vi "User Manage.vi"(11 "Name(\"\" to use uuid)":string="User Manage") -> ()   [LabVIEW 2020]
uses:
  <userlib>/_NEVSTOP/Communicable State Machine(CSM)/_Support/Priority Queue/Priority Queue.lvclass/Priority Queue.ctl
  <userlib>/_NEVSTOP/Communicable State Machine(CSM)/_Polymophic/Build Register Status Message.vi
  4963c333-465a-4436-b278-b1f160975599.vi
  7cf3f4c3-14bd-4f57-b2e5-d8e33bc96a06.vi
  95563834-bb2d-4c57-ba94-2bf903f692ff.vi
  <userlib>/_NEVSTOP/Communicable State Machine(CSM)/_Support/Process/CSMP-Async Call.vi
  <userlib>/_NEVSTOP/Communicable State Machine(CSM)/_Support/GlobalEvent/GEvt-Generate Status Log.vi
  <userlib>/_NEVSTOP/Communicable State Machine(CSM)/_Support/Process/CSMP-Broadcast.vi
  <userlib>/_NEVSTOP/Communicable State Machine(CSM)/_Support/GlobalEvent/GEvt-Generate Interrupt Log.vi
  <userlib>/_NEVSTOP/Communicable State Machine(CSM)/_Support/GlobalEvent/GEvt-Generate Register Log.vi
  <userlib>/_NEVSTOP/Communicable State Machine(CSM)/_Support/Process/CSMP-Register Status.vi
  <userlib>/_NEVSTOP/Communicable State Machine(CSM)/_Support/GlobalEvent/GEvt-Generate Unregister Log.vi
  <userlib>/_NEVSTOP/Communicable State Machine(CSM)/_Support/Process/CSMP-Unregister Status.vi
  <userlib>/_NEVSTOP/Communicable State Machine(CSM)/_Support/Process/CSMP-Sync Call.vi
  <userlib>/_NEVSTOP/Communicable State Machine(CSM)/_Support/CSMQ/_CSMObj-Unlock.vi
  <userlib>/_NEVSTOP/Communicable State Machine(CSM)/_Support/Process/CSMP-PostPostMsg.vi
  <userlib>/_NEVSTOP/Communicable State Machine(CSM)/_Support/Process/CSMP-PostSendMsg.vi
  <userlib>/_NEVSTOP/Communicable State Machine(CSM)/_Support/CSMQ/_CSMObj-Lock State.vi
  <userlib>/_NEVSTOP/Communicable State Machine(CSM)/_Support/Common/Splite Reason String Part.vi
  <userlib>/_NEVSTOP/Communicable State Machine(CSM)/_Support/Common/Trim Single line Text.vi
  <userlib>/_NEVSTOP/Communicable State Machine(CSM)/_Support/CSMQ/_CSMOFGV Release.vi
  <userlib>/_NEVSTOP/Communicable State Machine(CSM)/_Support/Common/Remove Comments from Line.vi
  <userlib>/_NEVSTOP/Communicable State Machine(CSM)/_Support/Common/Splite Single-line Message.vi
  <userlib>/_NEVSTOP/Communicable State Machine(CSM)/_Support/Common/Parse Next Single-line State.vi
  <userlib>/_NEVSTOP/Communicable State Machine(CSM)/_Support/CSMQ/_CSMOFGV Dequeue.vi
  <userlib>/_NEVSTOP/Communicable State Machine(CSM)/_Support/CSMQ/_CSMObj-Log Error if in a Remote Session.vi
  <userlib>/_NEVSTOP/Communicable State Machine(CSM)/_Support/GlobalEvent/GEvt-Generate State Change Log.vi
  <userlib>/_NEVSTOP/Communicable State Machine(CSM)/_Support/GlobalEvent/GEvt-Generate Remaining States Log.vi
  <userlib>/_NEVSTOP/Communicable State Machine(CSM)/_Support/GlobalEvent/GEvt-Generate Module Destroyed Log.vi
  <userlib>/_NEVSTOP/Communicable State Machine(CSM)/_Support/GlobalEvent/GEvt-Generate Complete Log.vi
  <userlib>/_NEVSTOP/Communicable State Machine(CSM)/_Support/GlobalEvent/GEvt-Generate Module Created Log.vi
  <userlib>/_NEVSTOP/Communicable State Machine(CSM)/_Support/GlobalEvent/Cache-GEvt Filter Object.vi
  <userlib>/_NEVSTOP/Communicable State Machine(CSM)/_Support/Common/Format Timestamp.vi
  <userlib>/_NEVSTOP/Communicable State Machine(CSM)/AdvanceAPI/CSM - Revert Arguments-Safe String.vi
  <userlib>/_NEVSTOP/Communicable State Machine(CSM)/AdvanceAPI/CSM - Make String Arguments Safe.vi
  <userlib>/_NEVSTOP/Communicable State Machine(CSM)/AdvanceAPI/CSM - Break Down Multiple States String.vi
  <userlib>/_NEVSTOP/Communicable State Machine(CSM)/AdvanceAPI/CSM - Compact Multiple States.vi
  <userlib>/_NEVSTOP/Communicable State Machine(CSM)/Utility/Trim Both Whitespace.vi
  <userlib>/_NEVSTOP/Communicable State Machine(CSM)/_Support/CSMQ/_CSMObj-Message Check.vi
  <userlib>/_NEVSTOP/Communicable State Machine(CSM)/_Support/CSMQ/_CSMObj-Enqueue Cross-Module Message.vi
  <userlib>/_NEVSTOP/Communicable State Machine(CSM)/_Support/CSMQ/_CSMOFGV Get.vi
  <userlib>/_NEVSTOP/Communicable State Machine(CSM)/_Support/GlobalEvent/GEvt-Generate with Rule Check.vi
  <userlib>/_NEVSTOP/Communicable State Machine(CSM)/_Support/FGV-BroadcastRegistry/Cache-Broadcast Registry Search Result.vi
  <userlib>/_NEVSTOP/Communicable State Machine(CSM)/AdvanceAPI/CSM - Register Status Change.vi
  <userlib>/_NEVSTOP/Communicable State Machine(CSM)/AdvanceAPI/CSM - Unregister Status Change.vi
  <userlib>/_NEVSTOP/Communicable State Machine(CSM)/_Support/Common/Hex Str to U8 Data.vi
  <userlib>/_NEVSTOP/Communicable State Machine(CSM)/_Support/Common/Concatenate State with Arguments.vi
  <userlib>/_NEVSTOP/Communicable State Machine(CSM)/_Support/Common/U8 Data to Hex Str.vi
  <userlib>/_NEVSTOP/Communicable State Machine(CSM)/_Support/Priority Queue/Dequeue Element.vi
  <userlib>/_NEVSTOP/Communicable State Machine(CSM)/AdvanceAPI/CSM - Keywords.vi
  <userlib>/_NEVSTOP/Communicable State Machine(CSM)/_Support/Priority Queue/Enqueue Element.vi
  <userlib>/_NEVSTOP/Communicable State Machine(CSM)/_Support/GlobalEvent/LogFilter/Filter Check.vi
  <userlib>/_NEVSTOP/Communicable State Machine(CSM)/_Support/GlobalEvent/FGV-GlobalEventRef.vi
  <userlib>/_NEVSTOP/Communicable State Machine(CSM)/_Support/GlobalEvent/global-GEvnt Filter Change Flag.vi
  <userlib>/_NEVSTOP/Communicable State Machine(CSM)/FGV-GEvt Filter Obj.vi
  <userlib>/_NEVSTOP/Communicable State Machine(CSM)/_Support/CSMQ/_CSMOFGV Obtain.vi
  <userlib>/_NEVSTOP/Communicable State Machine(CSM)/_Support/GlobalEvent/LogFilter/CheckVIs/Group Check - CSM.vi
  <userlib>/_NEVSTOP/Communicable State Machine(CSM)/_Support/GlobalEvent/LogFilter/CheckVIs/Group Check - LogType.vi
  <userlib>/_NEVSTOP/Communicable State Machine(CSM)/_Support/GlobalEvent/LogFilter/CheckVIs/Group Check - State.vi
  <userlib>/_NEVSTOP/Communicable State Machine(CSM)/_Support/GlobalEvent/LogFilter/CheckVIs/CSM Check - LogType.vi
  <userlib>/_NEVSTOP/Communicable State Machine(CSM)/_Support/GlobalEvent/LogFilter/CheckVIs/CSM Check - State.vi
  <userlib>/_NEVSTOP/Communicable State Machine(CSM)/_Support/GlobalEvent/LogFilter/CheckVIs/CSM Check - StateType.vi
  <userlib>/_NEVSTOP/Communicable State Machine(CSM)/_Support/GlobalEvent/LogFilter/CheckVIs/Group Check - StateType.vi
  <userlib>/_NEVSTOP/Communicable State Machine(CSM)/_Support/CSMQ/_CSMOFGV.vi
  <userlib>/_NEVSTOP/Communicable State Machine(CSM)/_Support/Error/CSM Not Allowed Message.vi
  <userlib>/_NEVSTOP/Communicable State Machine(CSM)/_Support/GlobalEvent/FGV-StatusChangeEventRef.vi
  <userlib>/_NEVSTOP/Communicable State Machine(CSM)/_Support/FGV-BroadcastRegistry/global-CSMQ FGV Change Flag.vi
  <userlib>/_NEVSTOP/Communicable State Machine(CSM)/_Support/FGV-BroadcastRegistry/global-Broadcast Cache Change Flag.vi
  <userlib>/_NEVSTOP/Communicable State Machine(CSM)/_Support/BroadcastRegistry/HelperVI/Broadcast Item Key.vi
  <userlib>/_NEVSTOP/Communicable State Machine(CSM)/_Support/FGV-BroadcastRegistry/FGV-BroadcastRegistry.vi
  <userlib>/_NEVSTOP/Communicable State Machine(CSM)/_Support/Message/Parse Register Message.vi
  <userlib>/_NEVSTOP/Communicable State Machine(CSM)/_Support/Message/Parse Unregister Message.vi
  <userlib>/_NEVSTOP/Communicable State Machine(CSM)/addons/API-String-Arugments-Support/_Support/Convert API String Arguments to Data(variant).vi
  <vilib>/Utility/config.llb/Read Key (String).vi
  <vilib>/Utility/config.llb/Write Key (String).vi
  <userlib>/_NEVSTOP/Communicable State Machine(CSM)/addons/API-String-Arugments-Support/_Support/Data To API String Arguments.vi
  <userlib>/_NEVSTOP/Communicable State Machine(CSM)/Communicable State Machine.lvlib
  <vilib>/Utility/config.llb/NI_LVConfig.lvlib
panel:
  out "Error Occurred":errorcluster
  out "State History":string
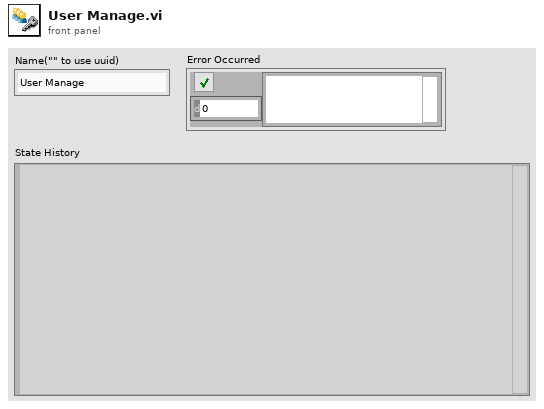
[diagram p1: front panel]
types:
  T1 = enum32{"Invalid", "Standard", "Closed", "Hidden", "Minimized", "Maximized"}
  T2 = enum32{"invalid app kind", "Development System", "Run Time System", "Student Edition", "Embedded LabVIEW", "Evaluation", "Custom"}
  T3 = typedef "Communicable State Machine.lvlib/_CSM_Response Source Message.ctl" = cluster{"‘State":string, "’Arguments":string, "’Error":errorcluster}
  T4 = cluster{"Current VI Reference":refnum<vi>, "Close Panel on Exit?":bool}
  T5 = cluster{"Core":cluster{"Current VI Reference":refnum<vi>, "Close Panel on Exit?":bool}, "Your Boolean data":bool, "ID":cluster{"password ":string, "username ":string}, "appended path":path}
  T6 = typedef "NI_LVConfig.lvlib/Config Data RefNum.ctl" = refnum<k1>
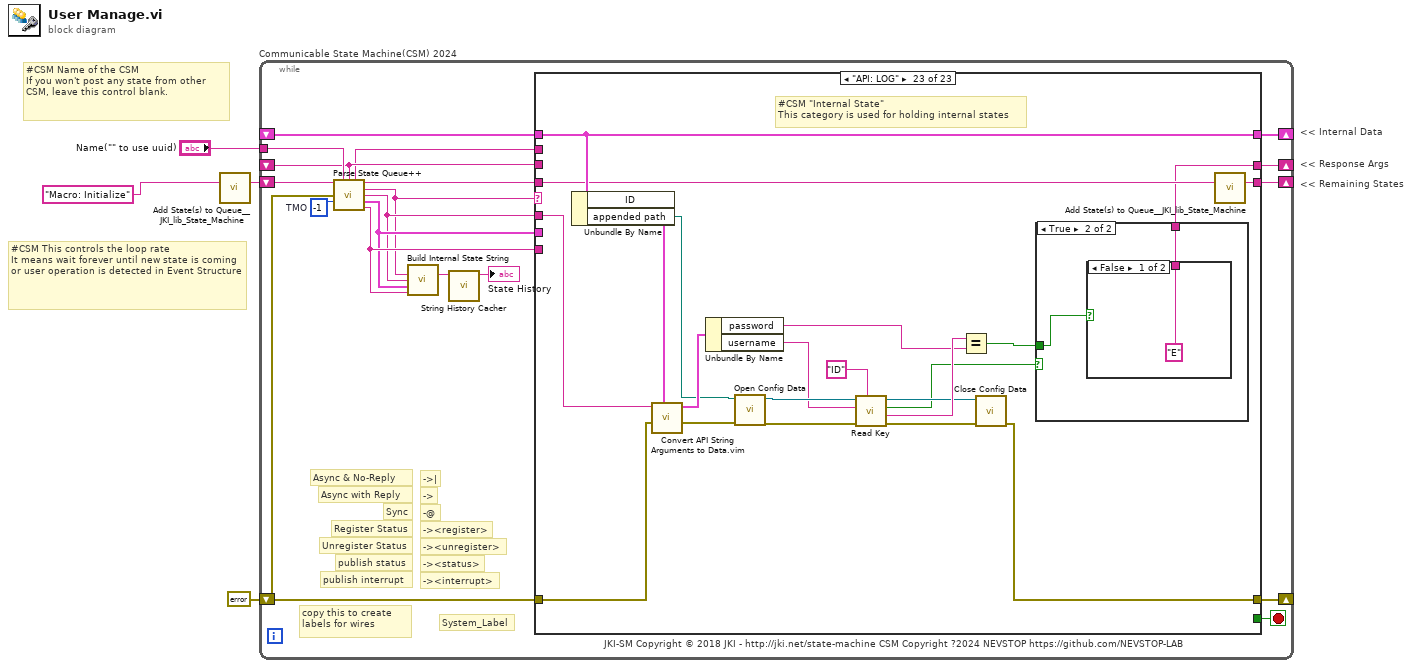
[diagram p0: block diagram]
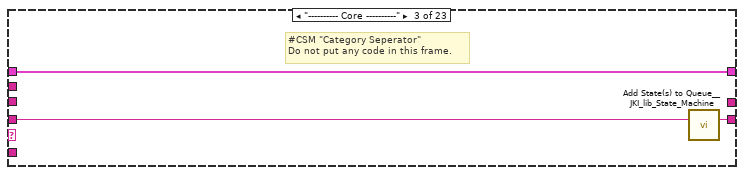
[diagram p4: hidden frame]
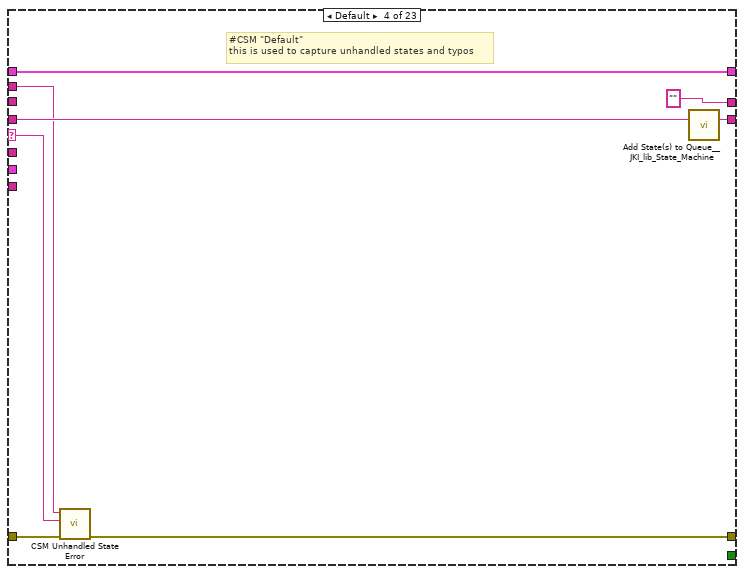
[diagram p5: hidden frame]
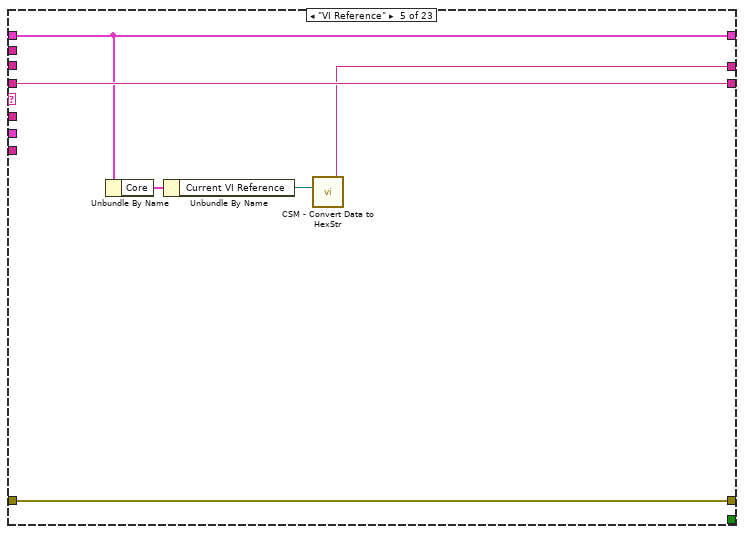
[diagram p6: hidden frame]
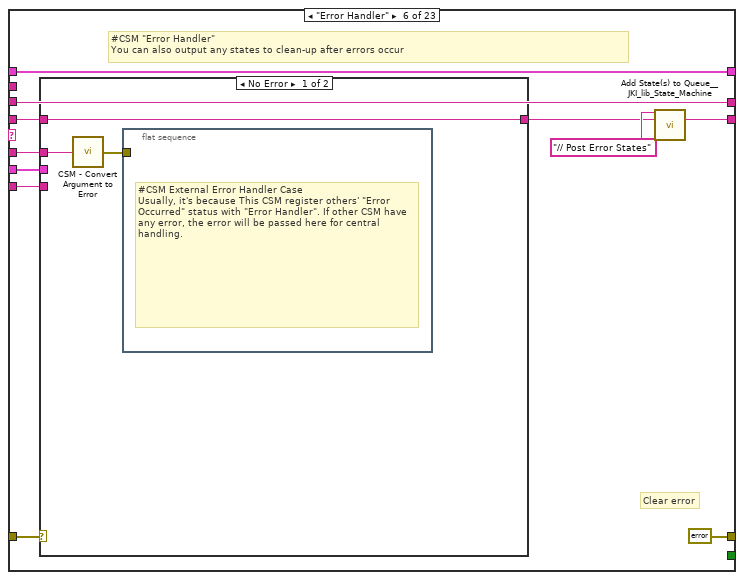
[diagram p7: hidden frame]
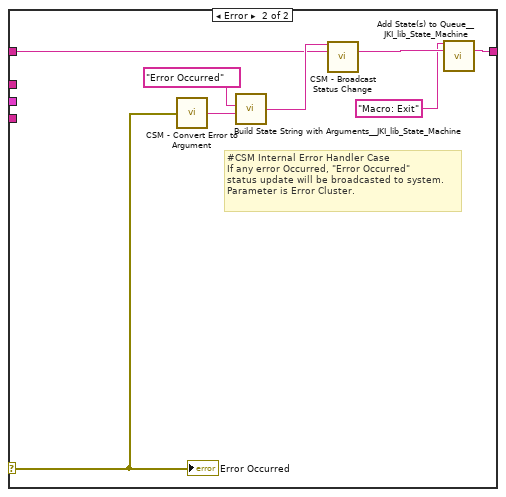
[diagram p8: hidden frame]
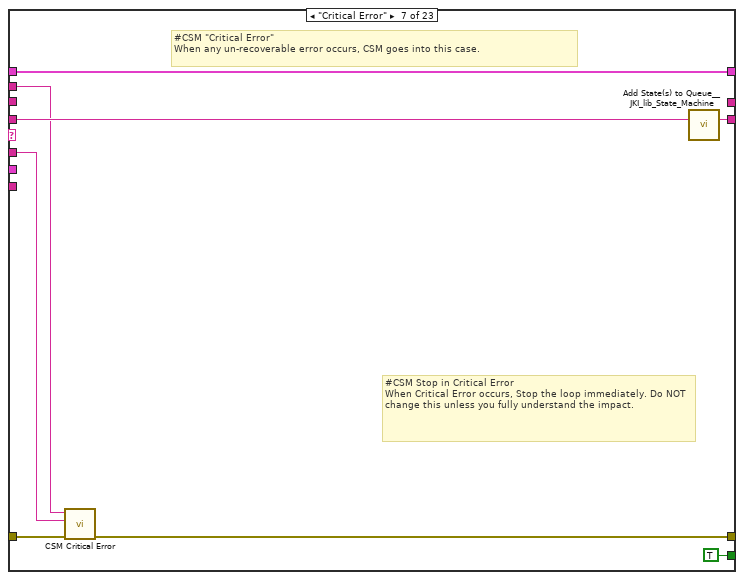
[diagram p9: hidden frame]
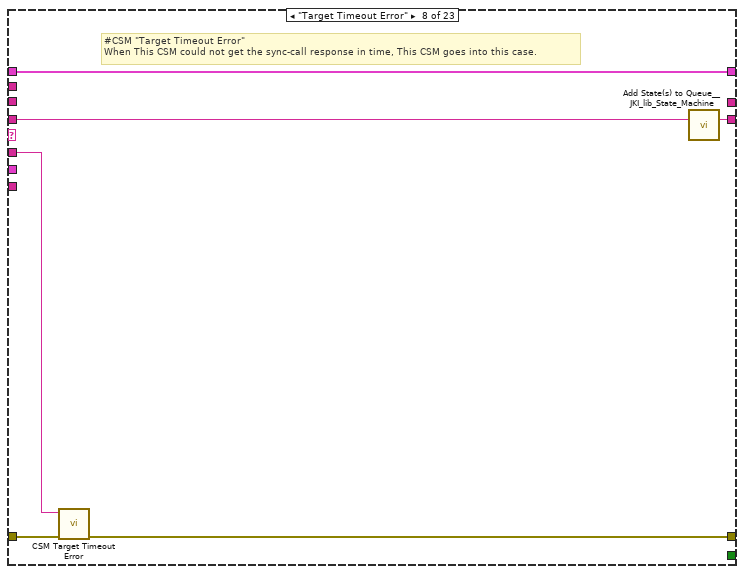
[diagram p10: hidden frame]
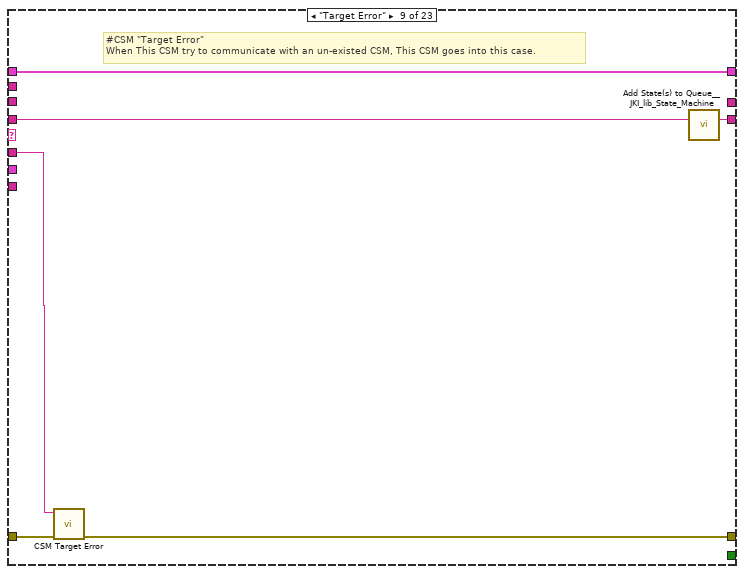
[diagram p11: hidden frame]
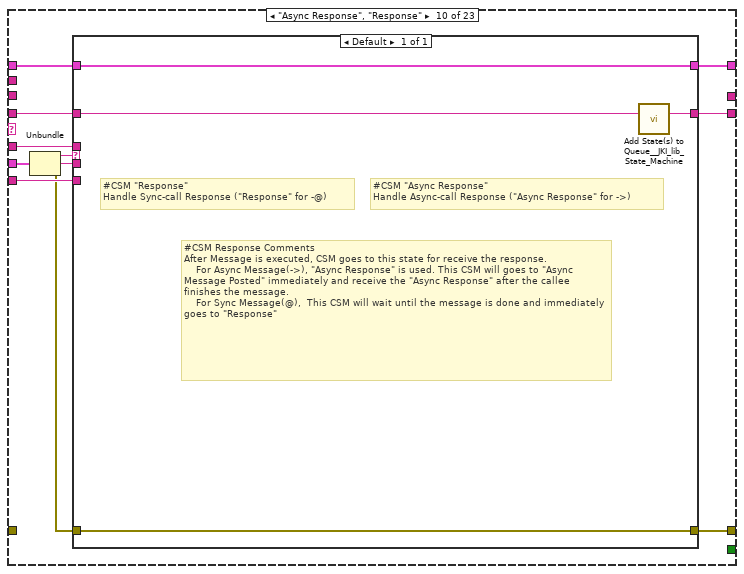
[diagram p12: hidden frame]
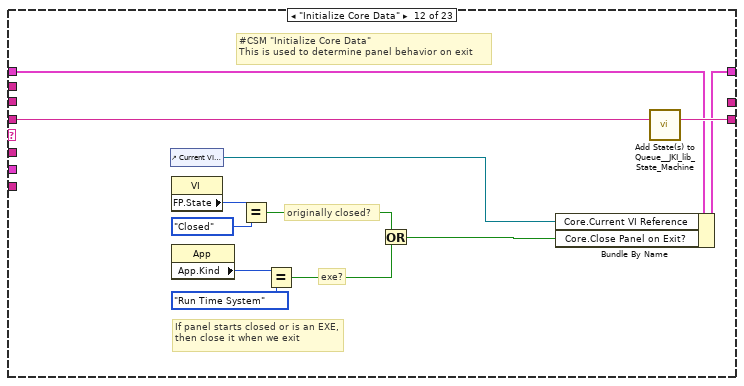
[diagram p14: hidden frame]
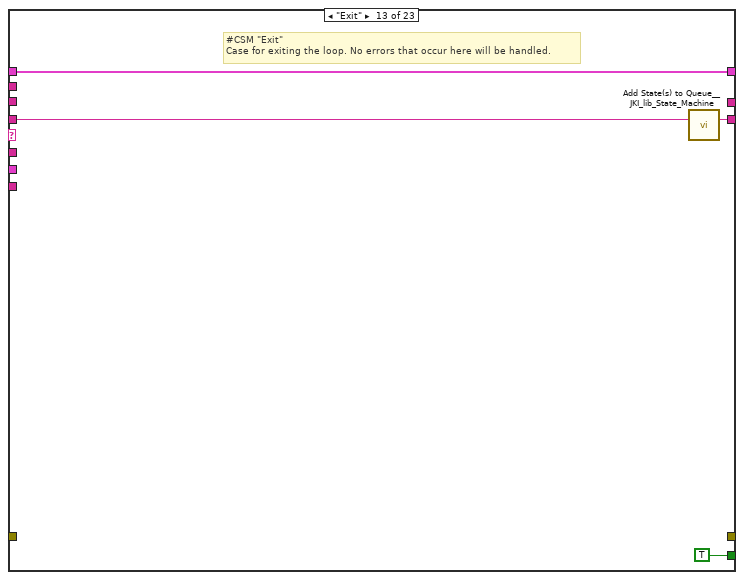
[diagram p15: hidden frame]
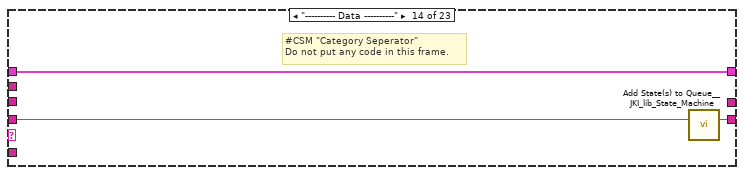
[diagram p16: hidden frame]
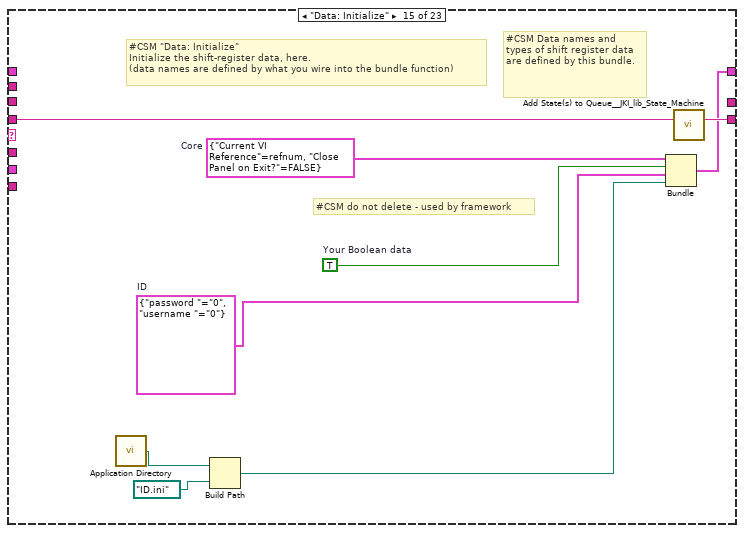
[diagram p17: hidden frame]
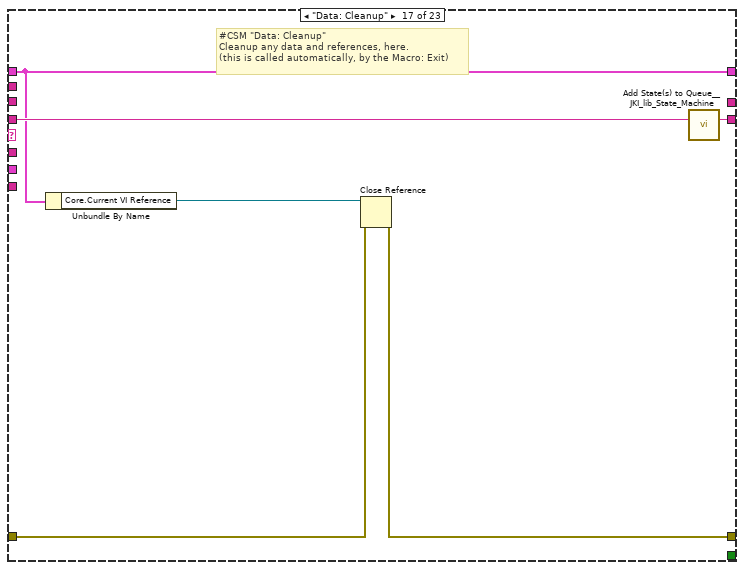
[diagram p19: hidden frame]
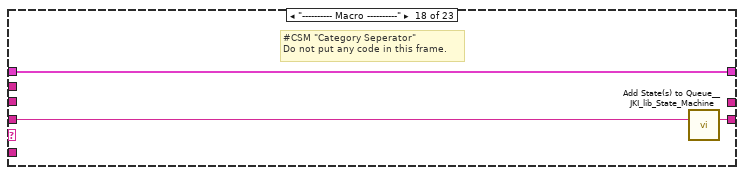
[diagram p20: hidden frame]
diagram:
  # "#CSM Name of the CSM\nIf you won't post any state from other CSM, leave this control blank."
  # "#CSM This controls the loop rate\nIt means wait forever until new state is coming or user operation is detected in Event Structure"
  # "<< Internal Data"
  # "<< Response Args"
  # "<< Remaining States"
  n1 = call <vilib>:"Add State(s) to Queue__JKI_lib_State_Machine.vi"("State(s) in (\"\")"="Macro: Initialize" ("Init State(\"Macro: Initialize\")")) -> ("States Out"=w2:string)  [unwired: 14 in]
  n2 = while "Communicable State Machine(CSM) 2024" {
    shift-right: [w18] -> _
    shift-left: _ -> [w17]
    shift-right: [w21] -> _
    shift-left: errorcluster {"status"=FALSE, "code"=0, "source"=""} ("error out") -> [w5]
    shift-right: [w20] -> _
    shift-left: w2 -> [w22]
    tunnel: "Name(\"\" to use uuid)" -> [w14]
    shift-right: [w15] -> _
    shift-left: _ -> [w7]
    stop <- w19 stop-if-true
    w16 = -1  # TMO
    # "-><interrupt>"
    # "-><status>"
    # "-><unregister>"
    # "-><register>"
    # "-@"
    # "->"
    # "->|"
    # "publish interrupt"
    # "publish status"
    # "Unregister Status"
    # "Register Status"
    # "Sync"
    # "Async with Reply"
    # "Async & No-Reply"
    # "JKI-SM Copyright © 2018 JKI - http://jki.net/state-machine CSM Copyright ?2024 NEVSTOP https://github.com/NEVSTOP-LAB"
    # "copy this to create labels for wires"
    # "System_Label"
    n3 = call <userlib>:"Parse State Queue++.vi"("State Queue"=w22, "Name(\"\" to use uuid)"=w14, "Response Arguments"=w7, "Error In (no error)"=w5, "Dequeue Timeout(0ms)"=w16) -> ("Name Used"=w6:string, "Remaining States"=w23:string, "Current State"=w8:string, "Arguments"=w9:string, ">> Response Source Message >>"=w10:T3, ">> Source CSM >>"=w11:string)  [unwired: 5 in]
    n4 = call <userlib>:"Build Internal State String.vi"("State"=w8, "Arguments (\"\")"=w9, ">> Response Source Message >>"=w10, "Source (\"\")"=w11) -> ("State with Arguments"=w12:string)  [unwired: 11 in]
    n5 = call <userlib>:"String History Cacher.vi"("String"=w12) -> ("String Cache"=→"State History":string)  [unwired: 10 in]
    n6 = case shown="\"API: LOG\"" w8 {
      selector: w8 -> [_ _ _ w34 _ _ _ _ _ _ _ _ _ _ _ _ _ _ _ _ _ _ _]
      tunnel: w23 -> [w24 w27 w30 w38 w43 w49 w74 w80 w86 w96 w103 w115 w119 w122 w131 w133 w139 w142 w148 w158 w160 w188 w228]
      tunnel: w9 -> [_ _ _ _ _ w48 w70 w77 w83 w90 _ _ _ _ _ _ _ _ _ _ _ w185 w227]
      tunnel: w17 -> [w25 w26 w28 w36 w42 w54 w72 w78 w84 w94 w102 w109 w117 w120 _ w132 w134 w140 w151 w156 w159 w186 w229]
      tunnel: [_ _ _ w31 w44 errorcluster {"status"=FALSE, "code"=0, "source"=""} ("error out") w67 w75 w81 w97 _ _ _ _ _ _ w135 _ _ _ _ w181 w218] -> w21
      tunnel: w5 -> [_ _ _ w32 w44 w52 w68 w76 w82 _ _ _ _ _ _ _ w136 _ _ _ _ w178 w216]
      tunnel: [w24 w27 w29 w37 w43 w50 w73 w79 w85 w95 w103 w114 w118 w121 w130 w133 w138 w141 w152 w157 w160 w187 w236] -> w20
      tunnel: [_ _ _ _ _ _ TRUE _ _ _ _ _ TRUE _ _ _ _ _ _ _ _ _ _] -> w19
      tunnel: [w25 w26 w28 w36 w42 w54 w72 w78 w84 w93 w102 w113 w117 w120 w129 w132 w134 w140 w151 w156 w159 w186 w229] -> w18
      tunnel: w11 -> [_ _ _ _ _ w47 _ _ _ w91 _ _ _ _ _ _ _ _ _ _ _ _ _]
      tunnel: w10 -> [_ _ _ _ _ w46 _ _ _ w92 _ _ _ _ _ _ _ _ _ _ _ _ _]
      tunnel: [_ _ _ "" w39 w45 _ _ _ _ _ _ _ _ _ _ _ _ _ _ _ w182 w220] -> w15
      tunnel: w6 -> [_ _ _ w33 _ _ w69 _ _ _ _ _ _ _ _ _ _ _ w143 _ _ _ _]
      tunnel: w7 -> [_ _ _ _ _ w45 _ _ _ _ _ _ _ _ _ _ _ _ _ _ _ _ _]
      frame "", "Idle" {
        # "#CSM \"Idle/Event Handler\"\nexecutes when the state queue is empty"
      }
      frame "CSM Documentation" {
        # "#CSM Documentation"
        # "#CSM State Syntax\n\n// Comment line, all text to the right of “//” will be ignored\n// Local Message Example\nDoSth: DoA >> Arguments\n\n// Sync Call Example\nAPI: xxxx >> Arguments -@ TargetModule\n\n// Async Call Example\nAPI: xxxx >> Arguments -> TargetModule\n\n// Async Call without Reply Example\nAPI: xxxx >> Arguments ->| TargetModule\n\n// Broadcast normal status:\nStatus >> StatusArguments  -><status>\n\n// Broadcast Interrupt status:\nInterrupt >> StatusArguments  -><interrupt>\n\n// Register Source Module's status to Handler Module\nStatus@Source Module >> Handler Module@Handler Module -><register>\n\n// Unegister Source Module's status\nStatus@Source Module >> Handler Module -><unregister>"
        # "#CSM README FIRST\n\nCommunicable State Machine(CSM) is a LabVIEW application framework that builds upon JKI State Machine(JKISM). It follows the pattern of JKISM and extends the keywords to describe message communication between modules, including concepts such as Sync-Message, Async-Message, Subscription/Unsubscription of status - essential elements for creating reusable code modules. For more information, please visit the CSM wiki: https://nevstop-lab.github.io/CSM-Wiki/\n\nFor instructions on JKI State Machine, visit: \n    http://jki.net/state-machine/\nFor information about CSM, visit: \n    https://github.com/NEVSTOP-LAB"
        # "#CSM \"Documentation\"\nCase for holding CSM Documenation"
      }
      frame "---------- Core ----------" {
        # "#CSM \"Category Seperator\"\nDo not put any code in this frame."
        n7 = call <vilib>:"Add State(s) to Queue__JKI_lib_State_Machine.vi"("State(s) in (\"\")"=w30) -> ("States Out"=w29:string)  [unwired: 14 in]
      }
      frame Default {
        # "#CSM \"Default\"\nthis is used to capture unhandled states and typos"
        n8 = call <userlib>:"CSM Unhandled State Error.vi"("error in (no error)"=w32, "Current State"=w34, "CSM Name"=w33) -> ("error out"=w31:errorcluster)  [unwired: 8 in]
        n9 = call <vilib>:"Add State(s) to Queue__JKI_lib_State_Machine.vi"("State(s) in (\"\")"=w38) -> ("States Out"=w37:string)  [unwired: 14 in]
      }
      frame "VI Reference" {
        n10 = Unbundle By Name(w42) -> ("Core"=w41:T4)
        n11 = Unbundle By Name(w41) -> ("Current VI Reference"=w40:refnum<vi>)
        n12 = call <userlib>:"CSM - Convert Data to HexStr.vi"("Variant"=w40) -> ("HEX String (0-9,A-F)"=w39:string)  [unwired: 8 in]
      }
      frame "Error Handler" {
        # "#CSM \"Error Handler\"\nYou can also output any states to clean-up after errors occur"
        # "Clear error"
        n13 = case shown="No Error" w52 {
          selector: w52 -> [_ w62]
          tunnel: [w58 w61] -> w51
          tunnel: w49 -> [w58 w63]
          tunnel: w48 -> [w57 _]
          tunnel: w47 -> [_ _]
          tunnel: w46 -> [_ _]
          frame No Error {
            n14 = call <userlib>:"CSM - Convert Argument to Error.vi"("Argument"=w57) -> ("error"=w56:errorcluster)  [unwired: 4 in]
            n15 = flat-sequence {
              tunnel: w56 -> [_]
              frame #0 {
                # "#CSM External Error Handler Case\nUsually, it's because This CSM register others' \"Error Occurred\" status with \"Error Handler\". If other CSM have any error, the error will be passed here for central handling."
              }
            }
          }
          frame Error {
            # "#CSM Internal Error Handler Case \nIf any error Occurred, \"Error Occurred\" \nstatus update will be broadcasted to system.\nParameter is Error Cluster."
            n16 = call <userlib>:"CSM - Convert Error to Argument.vi"("error in (no error)"=w62) -> ("Arguments"=w65:string)  [unwired: 4 in]
            n17 = call <vilib>:"Build State String with Arguments__JKI_lib_State_Machine.vi"("Arguments (\"\")"=w65, "State"="Error Occurred" ("Status with Arguments")) -> ("State with Arguments"=w64:string)  [unwired: 4 in]
            n18 = call <userlib>:"CSM - Broadcast Status Change.vi"("Status with Arguments"=w64, "State Queue"=w63) -> ("Remaining States"=w60:string)  [unwired: 13 in]
            n19 = call <vilib>:"Add State(s) to Queue__JKI_lib_State_Machine.vi"("State(s) in Front (\"\")"="Macro: Exit" ("State(s) in Front (\"\")"), "State(s) in (\"\")"=w60) -> ("States Out"=w61:string)  [unwired: 13 in]
            "Error Occurred" <- w62
          }
        }
        n20 = call <vilib>:"Add State(s) to Queue__JKI_lib_State_Machine.vi"("State(s) in Front (\"\")"="// Post Error States", "State(s) in (\"\")"=w51) -> ("States Out"=w50:string)  [unwired: 13 in]
      }
      frame "Critical Error" {
        # "#CSM \"Critical Error\"\nWhen any un-recoverable error occurs, CSM goes into this case."
        # "#CSM Stop in Critical Error\nWhen Critical Error occurs, Stop the loop immediately. Do NOT change this unless you fully understand the impact."
        n21 = call <userlib>:"CSM Critical Error.vi"("error in (no error)"=w68, "Arugments(as Reason)"=w70, "CSM Name"=w69) -> ("error out"=w67:errorcluster)  [unwired: 8 in]
        n22 = call <vilib>:"Add State(s) to Queue__JKI_lib_State_Machine.vi"("State(s) in (\"\")"=w74) -> ("States Out"=w73:string)  [unwired: 14 in]
      }
      frame "Target Timeout Error" {
        # "#CSM \"Target Timeout Error\"\nWhen This CSM could not get the sync-call response in time, This CSM goes into this case."
        n23 = call <userlib>:"CSM Target Timeout Error.vi"("error in (no error)"=w76, "Arguments(as CSM Name)"=w77) -> ("error out"=w75:errorcluster)  [unwired: 9 in]
        n24 = call <vilib>:"Add State(s) to Queue__JKI_lib_State_Machine.vi"("State(s) in (\"\")"=w80) -> ("States Out"=w79:string)  [unwired: 14 in]
      }
      frame "Target Error" {
        # "#CSM \"Target Error\"\nWhen This CSM try to communicate with an un-existed CSM, This CSM goes into this case."
        n25 = call <userlib>:"CSM Target Error.vi"("error in (no error)"=w82, "Arguments(as CSM Name)"=w83) -> ("error out"=w81:errorcluster)  [unwired: 9 in]
        n26 = call <vilib>:"Add State(s) to Queue__JKI_lib_State_Machine.vi"("State(s) in (\"\")"=w86) -> ("States Out"=w85:string)  [unwired: 14 in]
      }
      frame "Async Response", "Response" {
        n27 = Unbundle(w92) -> ("‘State"=w89:string, "’Arguments"=w88:string, "’Error"=w87:errorcluster)
        n28 = case shown="Default" w89 {
          tunnel: [w98] -> w95
          tunnel: w96 -> [w99]
          tunnel: [w101] -> w93
          tunnel: w94 -> [w101]
          tunnel: [w100] -> w97
          tunnel: w87 -> [w100]
          tunnel: w91 -> [_]
          tunnel: w90 -> [_]
          tunnel: w88 -> [_]
          frame Default {
            # "#CSM \"Async Response\"\nHandle Async-call Response (\"Async Response\" for ->)"
            # "#CSM \"Response\"\nHandle Sync-call Response (\"Response\" for -@)"
            # "#CSM Response Comments\nAfter Message is executed, CSM goes to this state for receive the response.\n    For Async Message(->), \"Async Response\" is used. This CSM will goes to \"Async Message Posted\" immediately and receive the \"Async Response\" after the callee finishes the message.\n    For Sync Message(@),  This CSM will wait until the message is done and immediately goes to \"Response\""
            n29 = call <vilib>:"Add State(s) to Queue__JKI_lib_State_Machine.vi"("State(s) in (\"\")"=w99) -> ("States Out"=w98:string)  [unwired: 14 in]
          }
        }
      }
      frame "Async Message Posted" {
        # "#CSM \"Async Message Posted\"\nAfter Async Message is posted (-> or ->| ), CSM goes to this state for post-action.\nYou can use Argument - State to tell which Async Message is called."
      }
      frame "Initialize Core Data" {
        # "#CSM \"Initialize Core Data\"\nThis is used to determine panel behavior on exit"
        # "originally closed?"
        # "exe?"
        # "If panel starts closed or is an EXE, then close it when we exit"
        n30 = control-ref of="Current VI Reference"() -> (w107:refnum<vi>)
        n31 = property class="VI"() -> ("FP.State"=w106:T1)  [unwired: 2 in, 2 out]
        n32 = property class="App"() -> ("App.Kind"=w112:T2)  [unwired: 2 in, 2 out]
        n33 = Equal?(x=w106, y=T1."Closed" ("Front Panel Window:State")) -> (x = y?=w104:bool)
        n34 = Equal?(x=w112, y=T2."Run Time System" ("Application:Kind")) -> (x = y?=w110:bool)
        n35 = Or(x=w104, y=w110) -> (x .or. y?=w108:bool)
        n36 = Bundle By Name(cluster=w109, "Core.Current VI Reference"=w107, "Core.Close Panel on Exit?"=w108) -> (w113:T5)
        n37 = call <vilib>:"Add State(s) to Queue__JKI_lib_State_Machine.vi"("State(s) in (\"\")"=w115) -> ("States Out"=w114:string)  [unwired: 14 in]
      }
      frame "Exit" {
        # "#CSM \"Exit\"\nCase for exiting the loop. No errors that occur here will be handled."
        n38 = call <vilib>:"Add State(s) to Queue__JKI_lib_State_Machine.vi"("State(s) in (\"\")"=w119) -> ("States Out"=w118:string)  [unwired: 14 in]
      }
      frame "---------- Data ----------" {
        # "#CSM \"Category Seperator\"\nDo not put any code in this frame."
        n39 = call <vilib>:"Add State(s) to Queue__JKI_lib_State_Machine.vi"("State(s) in (\"\")"=w122) -> ("States Out"=w121:string)  [unwired: 14 in]
      }
      frame "Data: Initialize" {
        w126 = cluster{"password ":string, "username ":string} {"password "="0", "username "="0"}  # ID
        w127 = T4 {"Current VI Reference"=refnum, "Close Panel on Exit?"=FALSE}  # Core
        w128 = TRUE  # Your Boolean data
        # "#CSM \"Data: Initialize\"\nInitialize the shift-register data, here.\n(data names are defined by what you wire into the bundle function)"
        # "#CSM do not delete - used by framework"
        # "#CSM Data names and types of shift register data are defined by this bundle."
        n40 = call <vilib>:"Application Directory.vi"() -> ("Application Directory"=w125:path)
        n41 = Build Path(base path=w125, name or relative path=path "ID.ini") -> (appended path=w123:path)
        n42 = Bundle("Core"=w127, "Your Boolean data"=w128, "ID"=w126, "appended path"=w123) -> (w129:T5)  [unwired: 1 in]
        n43 = call <vilib>:"Add State(s) to Queue__JKI_lib_State_Machine.vi"("State(s) in (\"\")"=w131) -> ("States Out"=w130:string)  [unwired: 14 in]
      }
      frame "Data: Update Indicators" {
      }
      frame "Data: Cleanup" {
        # "#CSM \"Data: Cleanup\"\nCleanup any data and references, here.\n(this is called automatically, by the Macro: Exit)"
        n44 = Unbundle By Name(w134) -> ("Core.Current VI Reference"=w137:refnum<vi>)
        n45 = Close Reference(reference=w137, error in (no error)=w136) -> (error out=w135:errorcluster)
        n46 = call <vilib>:"Add State(s) to Queue__JKI_lib_State_Machine.vi"("State(s) in (\"\")"=w139) -> ("States Out"=w138:string)  [unwired: 14 in]
      }
      frame "---------- Macro ----------" {
        # "#CSM \"Category Seperator\"\nDo not put any code in this frame."
        n47 = call <vilib>:"Add State(s) to Queue__JKI_lib_State_Machine.vi"("State(s) in (\"\")"=w142) -> ("States Out"=w141:string)  [unwired: 14 in]
      }
      frame "Macro: Initialize" {
        # "#CSM \"Macro: Initialize\"\nInitialization Macro (This is called once, when the VI starts)"
        n48 = call <vilib>:"Add State(s) to Queue__jki_lib_state_machine.vi"("State(s) in (\"\")"=w148) -> ("States Out"=w149:string)  [unwired: 14 in]
        n49 = call-poly <userlib>:"Build Message with Arguments++.vi"("CSM Name"=w143, "Source CSM Name (* as Default)"="*", "Status"="EXIT", "Response Message (if \"\", same as Source Message)"="Macro: Exit" ("Response Message (if \"\", same as Source Message)")) -> ("State with Arguments"=w144:string)  [unwired: 11 in]
        n50 = call <vilib>:"Add State(s) to Queue__JKI_lib_State_Machine.vi"("State(s) in Front (\"\")"="Data: Initialize\nInitialize Core Data\nData: Update Indicators", "State(s) in (\"\")"=w149, "State(s) at Back (\"\")"=w144) -> ("States Out"=w152:string)  [unwired: 12 in]
      }
      frame "Macro: Exit" {
        # "#CSM \"Macro: Exit\"\nExit Macro (This is called once, when the VI exits)"
        n51 = call <vilib>:"Add State(s) to Queue__JKI_lib_State_Machine.vi"("State(s) in Front (\"\")"="//Exit Sub-Modules ", "State(s) at Back (\"\")"="Data: Cleanup\nExit") -> ("States Out"=w154:string)  [unwired: 13 in]
        n52 = call <vilib>:"Add State(s) to Queue__JKI_lib_State_Machine.vi"("State(s) in Front (\"\")"=w154, "State(s) in (\"\")"=w158) -> ("States Out"=w157:string)  [unwired: 13 in]
      }
      frame "---------- API ----------" {
        # "#CSM \"Category Seperator\"\nDo not put any code in this frame."
      }
      frame "API: REG" {
        # "#CSM \"Internal State\"\nThis category is used for holding internal states"
        n53 = Unbundle By Name(w186) -> ("ID"=w179:cluster{"password ":string, "username ":string}, "appended path"=w183:path)
        n54 = call "Convert API String Arguments to Data.vim"("Type"=w179, "error in (no error)"=w178, "String"=w185) -> ("error"=w177:errorcluster, "Data"=w184:cluster{"password ":string, "username ":string})  [unwired: 5 in]
        n55 = Unbundle By Name(w184) -> ("username"=w161:string, "password"=w164:string)
        n56 = Match Pattern(string=w164, regular expression=" ") -> (match substring=w170:string)  [unwired: 1 in, 3 out]
        n57 = Match Pattern(string=w161, regular expression=" ") -> (match substring=w175:string)  [unwired: 1 in, 3 out]
        n58 = Empty String/Path?(string/path=w164) -> (empty?=w163:bool)
        n59 = Equal?(x=w170, y=" " ("regular expression")) -> (x = y?=w171:bool)
        n60 = Empty String/Path?(string/path=w161) -> (empty?=w162:bool)
        n61 = Equal?(x=w175, y=" " ("regular expression")) -> (x = y?=w173:bool)
        n62 = Or(x=w163, y=w171) -> (x .or. y?=w168:bool)
        n63 = Or(x=w162, y=w173) -> (x .or. y?=w167:bool)
        n64 = Or(x=w168, y=w167) -> (x .or. y?=w166:bool)
        n65 = case shown="True" w166 {
          tunnel: w183 -> [w195 _]
          tunnel: w161 -> [w193 _]
          tunnel: [w192 w215] -> w180
          tunnel: w164 -> [w191 _]
          tunnel: w177 -> [w190 w215]
          tunnel: [w189 "N"] -> w172
          frame False {
            n66 = call <vilib>:"Open Config Data.vi"("error in (no error)"=w190, "configuration file path"=w195) -> ("error out"=w199:errorcluster, "refnum"=w200:T6)  [unwired: 7 in, 1 out]
            n67 = call-poly <vilib>:"Read Key.vi"("section"="ID", "error in (no error)"=w199, "key"=w193, "refnum"=w200) -> ("error out"=w198:errorcluster, "found?"=w194:bool, "refnum out"=w197:T6)  [unwired: 4 in, 1 out]
            n68 = case shown="False" w194 {
              tunnel: [w204 w211] -> w192
              tunnel: w198 -> [w206 w212]
              tunnel: w197 -> [w209 w213]
              tunnel: w193 -> [w207 _]
              tunnel: w191 -> [w202 _]
              tunnel: ["Y" "E"] -> w189
              frame False {
                n69 = call-poly <vilib>:"Write Key.vi"("section"="ID", "error in (no error)"=w206, "value"=w202, "key"=w207, "refnum"=w209) -> ("error out"=w205:errorcluster, "refnum out"=w203:T6)  [unwired: 4 in, 1 out]
                n70 = call <vilib>:"Close Config Data.vi"("error in (no error)"=w205, "refnum"=w203) -> ("error out"=w204:errorcluster)  [unwired: 8 in, 1 out]
              }
              frame True {
                n71 = call <vilib>:"Close Config Data.vi"("error in (no error)"=w212, "refnum"=w213) -> ("error out"=w211:errorcluster)  [unwired: 8 in, 1 out]
              }
            }
          }
          frame True {
          }
        }
        n72 = call "Convert Data To API String Arguments.vim"("error in (no error)"=w180, "data"=w172) -> ("error out"=w181:errorcluster, "String"=w182:string)  [unwired: 6 in]
        n73 = call <vilib>:"Add State(s) to Queue__JKI_lib_State_Machine.vi"("State(s) in (\"\")"=w188) -> ("States Out"=w187:string)  [unwired: 14 in]
      }
      frame "API: LOG" {
        # "#CSM \"Internal State\"\nThis category is used for holding internal states"
        n74 = Unbundle By Name(w229) -> ("ID"=w226:cluster{"password ":string, "username ":string}, "appended path"=w222:path)
        n75 = call "Convert API String Arguments to Data.vim"("Type"=w226, "error in (no error)"=w216, "String"=w227) -> ("error"=w217:errorcluster, "Data"=w225:cluster{"password ":string, "username ":string})  [unwired: 5 in]
        n76 = Unbundle By Name(w225) -> ("password"=w223:string, "username"=w224:string)
        n77 = call <vilib>:"Open Config Data.vi"("error in (no error)"=w217, "configuration file path"=w222) -> ("error out"=w234:errorcluster, "refnum"=w235:T6)  [unwired: 7 in, 1 out]
        n78 = call-poly <vilib>:"Read Key.vi"("section"="ID", "error in (no error)"=w234, "key"=w224, "refnum"=w235) -> ("error out"=w232:errorcluster, "value"=w233:string, "found?"=w219:bool, "refnum out"=w231:T6)  [unwired: 4 in]
        n79 = Equal?(x=w233, y=w223) -> (x = y?=w221:bool)
        n80 = call <vilib>:"Close Config Data.vi"("error in (no error)"=w232, "refnum"=w231) -> ("error out"=w218:errorcluster)  [unwired: 8 in, 1 out]
        n81 = case shown="True" w219 {
          tunnel: w221 -> [_ w238]
          tunnel: ["N" ("String") w239] -> w220
          frame False {
          }
          frame True {
            n82 = case shown="False" w238 {
              tunnel: ["E" ("String") "Y" ("section")] -> w239
              frame False {
              }
              frame True {
              }
            }
          }
        }
        n83 = call <vilib>:"Add State(s) to Queue__JKI_lib_State_Machine.vi"("State(s) in (\"\")"=w228) -> ("States Out"=w236:string)  [unwired: 14 in]
      }
    }
  }
